vi "resetAllHP.vi"(8 "error in (no error)":errorcluster, 9 "TriggerIRQ":bool, 10 "WaitForTrigger":bool, 11 "ILCCommunications in":refnum<class "ILCCommunications.lvclass">) -> (0 "error out":errorcluster, 3 "ILCCommunications out":refnum<class "ILCCommunications.lvclass">)   [LabVIEW 2016, in "ILCCommunications.lvclass"]
uses:
  ILCCommunications.lvclass
  ILCCommunications.lvclass/ILCCommunications.ctl
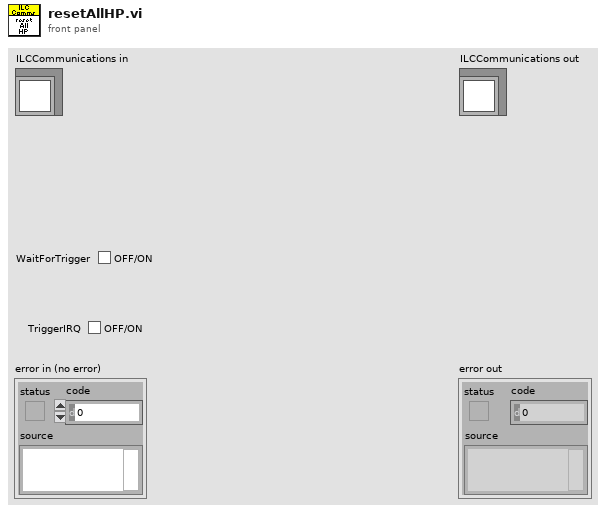
[diagram p1: front panel]
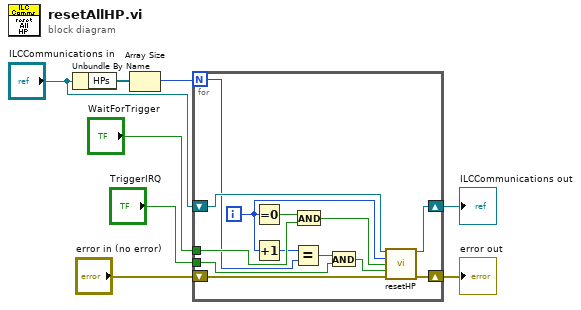
[diagram p0: block diagram]
diagram:
  n1 = Unbundle By Name("ILCCommunications in") -> ("HPs"=w8:refnum<class "HPILC.lvclass">[])
  n2 = Array Size(array=w8) -> (size(s)=w6:i32)
  n3 = for {
    N: w6 -> [w14]
    tunnel: "WaitForTrigger" -> [w17]
    tunnel: "TriggerIRQ" -> [w12]
    shift-right: [w19] -> w3
    shift-left: "ILCCommunications in" -> [w21]
    shift-right: [w20] -> w1
    shift-left: "error in (no error)" -> [w10]
    i -> [w9]
    n4 = Equal To 0?(x=w9) -> (x = 0?=w18:bool)
    n5 = Increment(x=w9) -> (x+1=w15:i32)
    n6 = Equal?(x=w15, y=w14) -> (x = y?=w13:bool)
    n7 = And(x=w18, y=w17) -> (x .and. y?=w16:bool)
    n8 = And(x=w13, y=w12) -> (x .and. y?=w11:bool)
    n9 = call "resetHP.vi"("ILCCommunications in"=w21, "HPIndex"=w9, "WaitForTrigger"=w16, "TriggerIRQ"=w11, "error in (no error)"=w10) -> ("ILCCommunications out"=w19:refnum<class "ILCCommunications.lvclass">, "error out"=w20:errorcluster)  [unwired: 9 in]
  }
  "error out" <- w1
  "ILCCommunications out" <- w3
